vi "string_to_path.vi"() -> ()   [LabVIEW 2021]
panel:
  out "file name":string
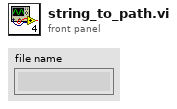
[diagram p1: front panel]
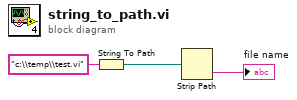
[diagram p0: block diagram]
diagram:
  n1 = String To Path(string="c:\\temp\\test.vi") -> (path=w3:path)
  n2 = Strip Path(path=w3) -> (name=→"file name":string)  [unwired: 1 out]
